vi "ORS-PathAddTimestamp.vi"(10 "timestamp?":bool=TRUE, 11 "path":path=path "c:/test.dat") -> (3 "path output":path=path "c:/2014.11.27_12.37.46_test.dat")   [LabVIEW 2024]
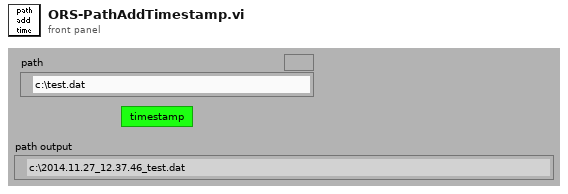
[diagram p1: front panel]
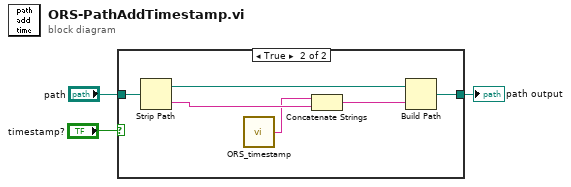
[diagram p0: block diagram]
diagram:
  n1 = case shown="True" "timestamp?" {
    tunnel: "path" -> [w4 w9]
    tunnel: [w4 w5] -> w1
    frame False {
    }
    frame True {
      n2 = Strip Path(path=w9) -> (stripped path=w8:path, name=w7:string)
      n3 = call "ORS_timestamp.vi"() -> ("system time"=w6:string)
      n4 = Concatenate Strings(w6, w7) -> (w10:string)
      n5 = Build Path(base path=w8, name or relative path=w10) -> (appended path=w5:path)
    }
  }
  "path output" <- w1
